vi "LED_Load Current Limit.vi"(0 "Set LED Current Limit?":bool, 5 "Load Current Limit Range":string, 7 "LED Current (Io)":dbl, 9 "DUT Current Limit in":dbl, 11 "error in":errorcluster) -> (4 "Current Limit Range":dbl, 8 "Current Limit":dbl, 15 "error out":errorcluster)   [LabVIEW 2021, in "start-up.lvlib"]
uses:
  start-up.lvlib
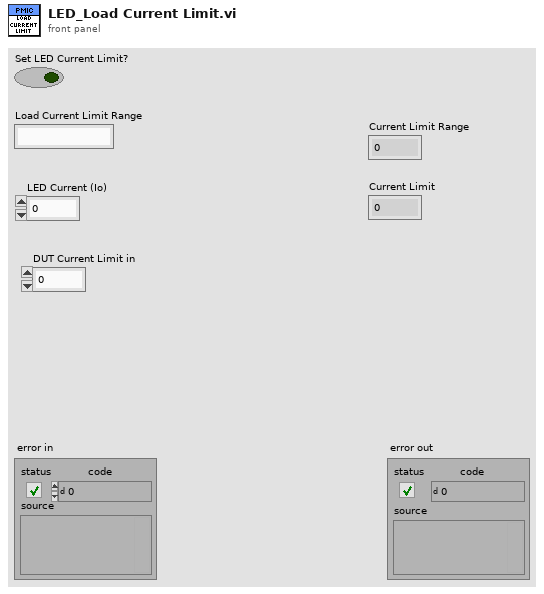
[diagram p1: front panel]
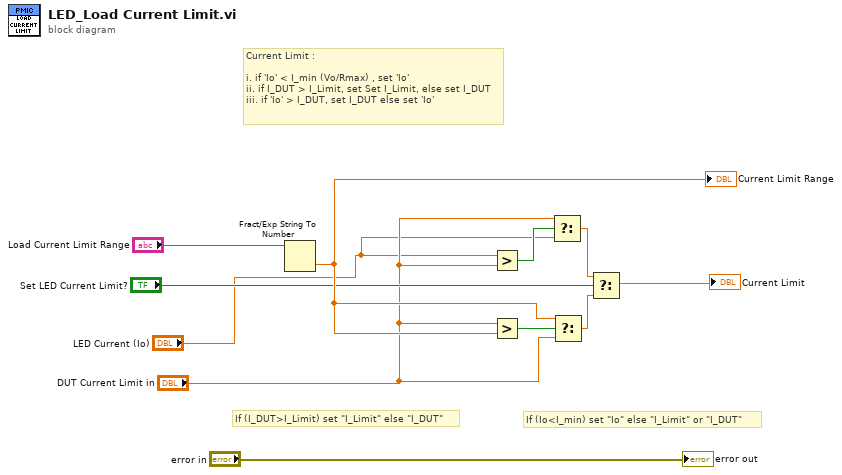
[diagram p0: block diagram]
diagram:
  # "If (I_DUT>I_Limit) set \"I_Limit\" else \"I_DUT\""
  # "If (Io<I_min) set \"Io\" else \"I_Limit\" or \"I_DUT\""
  # "Current Limit :\n\ni. if 'Io' < I_min (Vo/Rmax) , set 'Io'\nii. if I_DUT > I_Limit, set Set I_Limit, else set I_DUT\niii. if 'Io' > I_DUT, set I_DUT else set 'Io'"
  n1 = Fract/Exp String To Number(string="Load Current Limit Range") -> (number=w10:dbl)  [unwired: 3 in, 1 out]
  "Current Limit Range" <- w10
  n2 = Greater?(x="LED Current (Io)", y="DUT Current Limit in") -> (0:w5:bool)
  n3 = Greater?(x="DUT Current Limit in", y=w10) -> (0:w9:bool)
  n4 = Select(t="DUT Current Limit in", s=w5, f="LED Current (Io)") -> (s? t:f=w2:dbl)
  n5 = Select(t=w10, s=w9, f="DUT Current Limit in") -> (s? t:f=w11:dbl)
  n6 = Select(t=w2, s="Set LED Current Limit?", f=w11) -> (s? t:f=→"Current Limit":dbl)
  "error out" <- "error in"
